vi "Read Back a Slot Configuration.vi"() -> ()   [LabVIEW 2017]
uses:
  <vilib>/addons/VeriStand Custom Device Scripting APIs/Scan Engine/Modules/Mode Classes/Controls/counter driven output channel settings.ctl
  <vilib>/addons/VeriStand Custom Device Scripting APIs/Scan Engine/Modules/Channel Classes/Counter Driven Output Channel/Counter Driven State.ctl
  <vilib>/addons/VeriStand Custom Device Scripting APIs/Scan Engine/Modules/Mode Classes/Counter Driven Output Mode/Drive from Slot.ctl
  <vilib>/addons/VeriStand Custom Device Scripting APIs/Scan Engine/Scan Engine Dependencies.llb/Local Chassis Settings.ctl
  <vilib>/addons/VeriStand Custom Device Scripting APIs/Scan Engine/Scan Engine Dependencies.llb/Main Settings.ctl
  <vilib>/addons/VeriStand Custom Device Scripting APIs/Scan Engine/Modules/NI 9475/NI 9475.lvclass
  C:/Program Files (x86)/National Instruments/LabVIEW 2017/vi.lib/addons/VeriStand Custom Device Scripting APIs/Scan Engine/Modules/Module/Module.lvclass
  251745a7-ec8c-4a35-af18-abfda49c5109.vi
  <vilib>/addons/VeriStand Custom Device Scripting APIs/Scan Engine/Scan Engine Dependencies.llb/Set Error.vi
  <vilib>/Utility/error.llb/Clear Errors.vi
  <vilib>/addons/VeriStand Custom Device Scripting APIs/Scan Engine/Utility/Convert Slot Configuration to 9212.vi
  <vilib>/addons/VeriStand Custom Device Scripting APIs/Scan Engine/Utility/Convert Slot Configuration to 9213.vi
  <vilib>/addons/VeriStand Custom Device Scripting APIs/Scan Engine/Modules.lvlibp/SD Module/SD Module.lvclass
  C:/Program Files (x86)/National Instruments/LabVIEW 2017/vi.lib/addons/VeriStand Custom Device Scripting APIs/Scan Engine/Modules.lvlibp/RSI Module/RSI Module.lvclass
  <vilib>/addons/VeriStand Custom Device Scripting APIs/Scan Engine/Modules/NI 9212/NI 9212.lvclass
  <vilib>/addons/VeriStand Custom Device Scripting APIs/Scan Engine/Modules/NI 9213/NI 9213.lvclass
  <vilib>/addons/VeriStand Custom Device Scripting APIs/Scan Engine/Modules/NI 9224/NI 9224.lvclass
  <vilib>/addons/VeriStand Custom Device Scripting APIs/Scan Engine/Modules/NI 9228/NI 9228.lvclass
  <vilib>/addons/VeriStand Custom Device Scripting APIs/Scan Engine/Modules/NI 9475/Create NI 9475 - Counter Driven Output.vi
  <vilib>/addons/VeriStand Custom Device Scripting APIs/Scan Engine/Modules.lvlibp/RSI Module/Read Module Page Property.vi
  <vilib>/addons/VeriStand Custom Device Scripting APIs/Scan Engine/Modules.lvlibp/RSI Module/Read Model.vi
  <vilib>/addons/VeriStand Custom Device Scripting APIs/Scan Engine/Utility/Convert Module Model to Module Class.vi
  <vilib>/addons/VeriStand Custom Device Scripting APIs/Scan Engine/Modules.lvlibp/SD Module/Read DIO mode.vi
  <vilib>/addons/VeriStand Custom Device Scripting APIs/Scan Engine/Modules.lvlibp/RSI Module/Read Channels.vi
  <vilib>/addons/VeriStand Custom Device Scripting APIs/Scan Engine/Utility/Convert to DI Module.vi
  <vilib>/addons/VeriStand Custom Device Scripting APIs/Scan Engine/Utility/Convert to DO Module.vi
  <vilib>/addons/VeriStand Custom Device Scripting APIs/Scan Engine/Utility/Convert to CI PWM Module.vi
  <vilib>/addons/VeriStand Custom Device Scripting APIs/Scan Engine/Utility/Convert to CDO Module.vi
  <vilib>/addons/VeriStand Custom Device Scripting APIs/Scan Engine/Utility/Convert to PWM Module.vi
  <vilib>/addons/VeriStand Custom Device Scripting APIs/Scan Engine/Scan Engine Dependencies.llb/Error Strings.vi
  <vilib>/addons/VeriStand Custom Device Scripting APIs/Scan Engine/Utility/Get Channel Names and Default Values for Slot.vi
  <vilib>/addons/VeriStand Custom Device Scripting APIs/Scan Engine/Modules/NI 9212/Create NI 9212.vi
  <vilib>/addons/VeriStand Custom Device Scripting APIs/Scan Engine/Modules/NI 9213/Create NI 9213.vi
  <vilib>/addons/VeriStand Custom Device Scripting APIs/Scan Engine/Utility/Convert to AI Module.vi
  <vilib>/addons/VeriStand Custom Device Scripting APIs/Scan Engine/Utility/Convert to AI Vrms Module.vi
  <vilib>/addons/VeriStand Custom Device Scripting APIs/Scan Engine/Utility/Convert to AI Arms Module.vi
  <vilib>/addons/VeriStand Custom Device Scripting APIs/Scan Engine/Utility/Convert to DIO Module.vi
  <vilib>/addons/VeriStand Custom Device Scripting APIs/Scan Engine/Modules/NI 9475/Read NI 9475 - Counter Driven Output.vi
  <vilib>/addons/VeriStand Custom Device Scripting APIs/Scan Engine/Modules/Module/Module.lvclass
  <vilib>/addons/VeriStand Custom Device Scripting APIs/Scan Engine/Modules.lvlibp/9212/9212.lvclass
  <vilib>/addons/VeriStand Custom Device Scripting APIs/Scan Engine/Modules.lvlibp/9213/9213.lvclass
  <vilib>/addons/VeriStand Custom Device Scripting APIs/Scan Engine/Modules.lvlibp/9224/9224.lvclass
  SubVIs/Scan Engine Example Support.lvlib
  <vilib>/addons/VeriStand Custom Device Scripting APIs/Scan Engine/Scan Engine Scripting.lvlib
  <vilib>/addons/VeriStand Custom Device Scripting APIs/Scan Engine/Scan Engine Dependencies.llb/Scan Engine Custom Device.lvlib
  <vilib>/addons/VeriStand Custom Device Scripting APIs/Scan Engine/Modules/Mode Classes/Counter Driven Output Mode/Counter Driven Output Mode.lvclass
  <vilib>/addons/VeriStand Custom Device Scripting APIs/Scan Engine/Modules/Channel Classes/Counter Driven Output Channel/Counter Driven Output Channel.lvclass
panel:
  out "Drive From Slot":T1
  out "Channel Settings":T2[](array[typedef])
  in  "Input System Definition File":path=path "System Definition Files/Base.nivssdf"
  # "Overview: Demonstrates using the Scan Engine and EtherCAT scripting API to read a slot configuration from a system definition file that contains a Scan Engine Custom Device.\n\nInstructions:\n1. Browse to a system definition file to be used as the Input System Definition File that you would like to add a Scan Engine and EtherCAT custom device. This system defintion file should not already include a Scan Engine and EtherCAT custom device.\n2. Run the VI."
  # "System Definition File"
  # "Slot Properties"
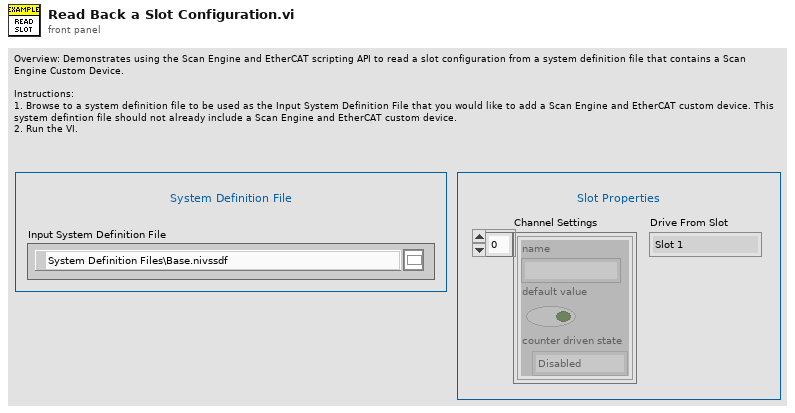
[diagram p1: front panel]
types:
  T1 = typedef "Scan Engine Scripting.lvlib/Counter Driven Output Mode.lvclass/Drive from Slot.ctl" = enum16{"Slot 1", "Slot 2", "Slot 3", "Slot 4", "Slot 5", "Slot 6", "Slot 7", "Slot 8"}
  T2 = typedef "Scan Engine Scripting.lvlib/counter driven output channel settings.ctl" = cluster{"name":string, "default value":bool, "counter driven state":T3}
  T3 = typedef "Scan Engine Scripting.lvlib/Counter Driven Output Channel.lvclass/Counter Driven State.ctl" = enum16{"Disabled", "Enabled"}
  T4 = typedef "Scan Engine Custom Device.lvlib/Main Settings.ctl" = cluster{"sync to scan":bool, "scan engine decimation":u16, "delay after FPGA load (s)":u16}
  T5 = typedef "Scan Engine Custom Device.lvlib/Local Chassis Settings.ctl" = cluster{"name":string, "number of slots":i32}
  T6 = typedef "Custom Device API.lvlib/Custom Device Item Ref.ctl" = u64
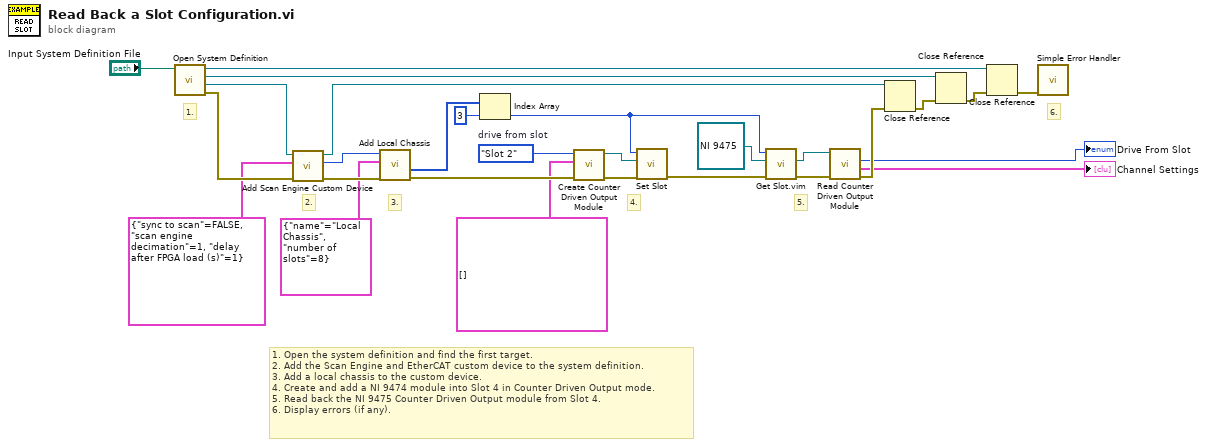
[diagram p0: block diagram]
diagram:
  w10 = Drive_from_Slot."Slot 2"  # drive from slot
  # "5."
  # "4."
  # "3."
  # "2."
  # "6."
  # "1."
  # "1. Open the system definition and find the first target.\n2. Add the Scan Engine and EtherCAT custom device to the system definition.\n3. Add a local chassis to the custom device.\n4. Create and add a NI 9474 module into Slot 4 in Counter Driven Output mode. \n5. Read back the NI 9475 Counter Driven Output module from Slot 4.\n6. Display errors (if any)."
  n1 = call "Open System Definition.vi"("System Definition File"="Input System Definition File") -> ("error out"=w20:errorcluster, "Target Refnum"=w22:refnum<k24>, "Root Refnum"=w27:refnum<k24>, "System Definition Refnum"=w28:refnum<k24>)  [unwired: 7 in]
  n2 = call <vilib>:"Add Scan Engine Custom Device.vi"("error in"=w20, "settings"=T4 {"sync to scan"=FALSE, "scan engine decimation"=1, "delay after FPGA load (s)"=1}, "target in"=w22) -> ("error out"=w18:errorcluster, "scan engine custom device ref"=w19:T6, "target out"=w21:refnum<k24>)  [unwired: 6 in]
  n3 = call <vilib>:"Add Local Chassis.vi"("error in"=w18, "settings"=T5 {"name"="Local Chassis", "number of slots"=8}, "scan engine custom device ref in"=w19) -> ("error out"=w17:errorcluster, "slot refs"=w14:T6[])  [unwired: 4 in, 3 out]
  n4 = Index Array(array=w14, index=3) -> (element=w7:T6)
  n5 = call-poly <vilib>:"Create Counter Driven Output Module.vi"("error in"=w17, "channel settings"=T2[] [], "drive from slot"=w10) -> ("error out"=w16:errorcluster, "NI 9475 out"=w15:refnum<class "NI 9475.lvclass">)  [unwired: 7 in]
  n6 = call <vilib>:"Set Slot.vi"("error in"=w16, "module"=w15, "slot ref in"=w7) -> ("error out"=w8:errorcluster)  [unwired: 7 in, 1 out]
  n7 = call "Get Slot.vim"("error in"=w8, "module in"=refnum<class "NI 9475.lvclass"> refnum ("NI 9475 out"), "slot ref in"=w7) -> ("error out"=w4:errorcluster, "module"=w5:refnum<class "NI 9475.lvclass">)  [unwired: 5 in, 2 out]
  n8 = call-poly <vilib>:"Read Counter Driven Output Module.vi"("error in"=w4, "NI 9475 in"=w5) -> ("error out"=w3:errorcluster, "channel settings"=→"Channel Settings":T2[], "drive from slot"=→"Drive From Slot":T1)  [unwired: 6 in, 1 out]
  n9 = Close Reference(reference=w21, error in (no error)=w3) -> (error out=w25:errorcluster)
  n10 = Close Reference(reference=w27, error in (no error)=w25) -> (error out=w26:errorcluster)
  n11 = Close Reference(reference=w28, error in (no error)=w26) -> (error out=w24:errorcluster)
  n12 = call <vilib>:"Simple Error Handler.vi"("error in (no error)"=w24) -> ()  [unwired: 1 in, 8 out]
